vi "Update.vi"(8 "error in (no error)":errorcluster, 11 "VacuumLine in":refnum<class "VacuumLine.lvclass">) -> (0 "error out":errorcluster, 3 "VacuumLine out":refnum<class "VacuumLine.lvclass">)   [LabVIEW 2016, in "Hardware.lvlib" / "VacuumLine.lvlib" / "VacuumLine.lvclass"]
uses:
  <userlib>/Common Components/Hardware/Abstract System/VacuumLine/VacuumLine/VacuumLine.lvclass
  <userlib>/Common Components/Hardware/Abstract System/VacuumLine/VacuumLine/VacuumLine.lvclass/VacuumLine.ctl
  <userlib>/Common Components/Hardware/Displacement Sensor/DispSnsr/DispSnsr.lvclass
  <userlib>/Common Components/Hardware/Motor/Motor/Motor.lvclass
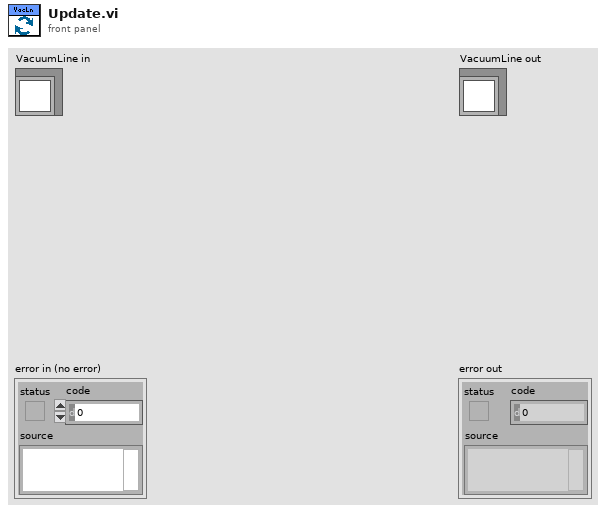
[diagram p1: front panel]
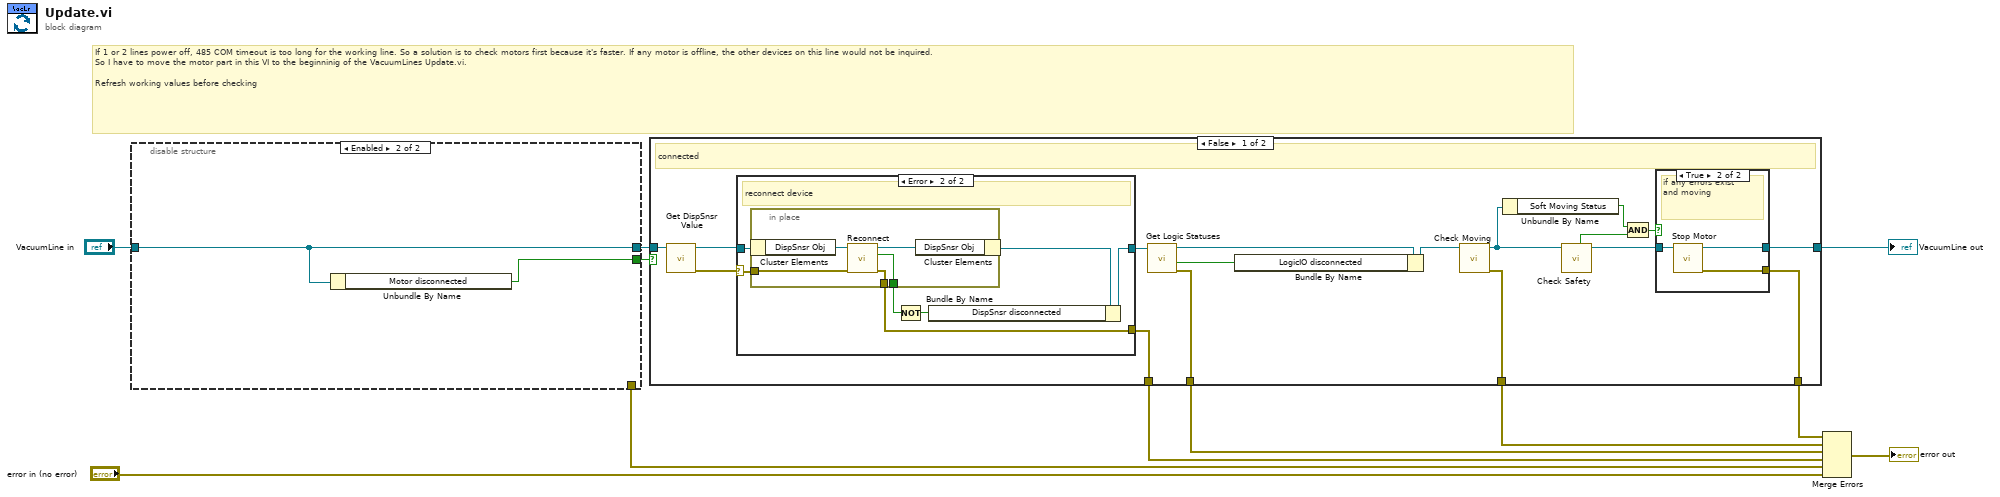
[diagram p0: block diagram]
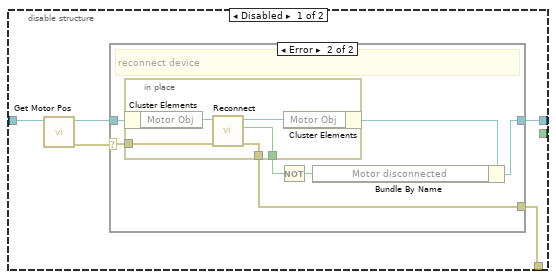
[diagram p5: hidden frame]
diagram:
  # "If 1 or 2 lines power off, 485 COM timeout is too long for the working line. So a solution is to check motors first because it's faster. If any motor is offline, the other devices on this line would not be inquired.\nSo I have to move the motor part in this VI to the beginninig of the VacuumLines Update.vi. \n\nRefresh working values before checking"
  n1 = disable-structure shown="Enabled" {
    disable-tunnel: "VacuumLine in" -> [w16 w32]
    disable-tunnel: [w14 w32] -> w7
    disable-tunnel: [w12 _] -> w3
    disable-tunnel: [_ w31] -> w1
    frame Disabled {
      n2 = call <userlib>:"Get Motor Pos.vi"("VacuumLine in"=w16) -> ("error out"=w13:errorcluster, "VacuumLine out"=w15:refnum<class "VacuumLine.lvclass">)  [unwired: 8 in, 1 out]
      n3 = case shown="Error" w13 {
        selector: w13 -> [w17 w21]
        tunnel: w15 -> [w18 w25]
        tunnel: [w18 w23] -> w14
        tunnel: [w17 w20] -> w12
        frame No Error {
        }
        frame Error {
          # "reconnect device"
          n4 = in-place {
            in-place-border: w21 -> [w28]
            in-place-border: [w27] -> w20
            in-place-border: [w26] -> w19
            n5 = in-place-cluster #1(w25) -> ("Motor Obj"=w30:refnum<class "Motor.lvclass">)
            n6 = call-dynamic "Reconnect.vi"("error in (With error)"=w28, "Hardware in"=w30) -> ("error out"=w27:errorcluster, "Reconnected"=w26:bool, "Hardware out"=w29:refnum<class "Motor.lvclass">)  [unwired: 7 in]
            n7 = in-place-cluster #1("Motor Obj"=w29) -> (w24:refnum<class "VacuumLine.lvclass">)
          }
          n8 = Not(x=w19) -> (.not. x?=w22:bool)
          n9 = Bundle By Name(cluster=w24, "Motor disconnected"=w22) -> (w23:refnum<class "VacuumLine.lvclass">)
        }
      }
    }
    frame Enabled {
      n10 = Unbundle By Name(w32) -> ("Motor disconnected"=w31:bool)
    }
  }
  n11 = case shown="False" w1 {
    tunnel: [w47 w68] -> w10
    tunnel: w7 -> [w45 w68]
    tunnel: [w42 _] -> w6
    tunnel: [w41 _] -> w5
    tunnel: [w40 _] -> w4
    tunnel: [w35 _] -> w2
    frame False {
      # "connected"
      n12 = call <userlib>:"Get DispSnsr Value.vi"("VacuumLine in"=w45) -> ("error out"=w39:errorcluster, "VacuumLine out"=w44:refnum<class "VacuumLine.lvclass">)  [unwired: 8 in, 1 out]
      n13 = case shown="Error" w39 {
        selector: w39 -> [w50 w54]
        tunnel: w44 -> [w51 w58]
        tunnel: [w51 w56] -> w43
        tunnel: [w50 w52] -> w35
        frame No Error {
        }
        frame Error {
          # "reconnect device"
          n14 = in-place {
            in-place-border: w54 -> [w60]
            in-place-border: [w61] -> w53
            in-place-border: [w59] -> w52
            n15 = in-place-cluster #2(w58) -> ("DispSnsr Obj"=w63:refnum<class "DispSnsr.lvclass">)
            n16 = call-dynamic "Reconnect.vi"("error in (With error)"=w60, "Hardware in"=w63) -> ("error out"=w59:errorcluster, "Reconnected"=w61:bool, "Hardware out"=w62:refnum<class "DispSnsr.lvclass">)  [unwired: 7 in]
            n17 = in-place-cluster #2("DispSnsr Obj"=w62) -> (w57:refnum<class "VacuumLine.lvclass">)
          }
          n18 = Not(x=w53) -> (.not. x?=w55:bool)
          n19 = Bundle By Name(cluster=w57, "DispSnsr disconnected"=w55) -> (w56:refnum<class "VacuumLine.lvclass">)
        }
      }
      n20 = call <userlib>:"Get Logic Statuses.vi"("VacuumLine in"=w43) -> ("error out"=w42:errorcluster, "disconnected"=w33:bool, "VacuumLine out"=w49:refnum<class "VacuumLine.lvclass">)  [unwired: 7 in, 1 out]
      n21 = Bundle By Name(cluster=w49, "LogicIO disconnected"=w33) -> (w34:refnum<class "VacuumLine.lvclass">)
      n22 = call <userlib>:"Check Moving.vi"("VacuumLine in"=w34) -> ("error out"=w41:errorcluster, "VacuumLine out"=w37:refnum<class "VacuumLine.lvclass">)  [unwired: 7 in, 2 out]
      n23 = Unbundle By Name(w37) -> ("Soft Moving Status"=w36:bool)
      n24 = call <userlib>:"Check Safety.vi"("VacuumLine in"=w37) -> ("VacuumLine out"=w48:refnum<class "VacuumLine.lvclass">, "Error"=w46:bool)  [unwired: 8 in, 1 out]
      n25 = And(x=w36, y=w46) -> (x .and. y?=w38:bool)
      n26 = case shown="True" w38 {
        tunnel: [_ w67] -> w40
        tunnel: w48 -> [w64 w66]
        tunnel: [w64 w65] -> w47
        frame False {
        }
        frame True {
          # "if any errors exist and moving"
          n27 = call <userlib>:"Stop Motor.vi"("VacuumLine in"=w66) -> ("error out"=w67:errorcluster, "VacuumLine out"=w65:refnum<class "VacuumLine.lvclass">)  [unwired: 9 in]
        }
      }
    }
    frame True {
      # "disconnected"
    }
  }
  "VacuumLine out" <- w10
  n28 = Merge Errors(w4, w5, w6, w2, w3, "error in (no error)") -> (→"error out":errorcluster)
